vi "Write Report.vi"(8 "error in (no error)":errorcluster, 10 "Resource In":variant, 11 "Analyze Parameter Spectral Calibration in":refnum<class "Analyze Parameter Spectral Calibration.lvclass">) -> (0 "error out":errorcluster, 2 "Resource Out":variant, 3 "Analyze Parameter Spectral Calibration out":refnum<class "Analyze Parameter Spectral Calibration.lvclass">)   [LabVIEW 2020, in "Analyze Parameter Spectral Calibration.lvclass"]
uses:
  Analyze Parameter Spectral Calibration.lvclass
  C:/POLARIS Programme/POLARIS-AS-3-Cams/Submodules/HIJ Vision/Analyze/Analyze Parameter/Analyze Parameter Base/Analyze Parameter Base.lvclass
  <vilib>/Utility/config.llb/Config Data RefNum.ctl
  Analyze Parameter Spectral Calibration.lvclass/Analyze Parameter Spectral Calibration.ctl
  <vilib>/Utility/config.llb/Write Key (Double).vi
  <vilib>/Utility/config.llb/NI_LVConfig.lvlib
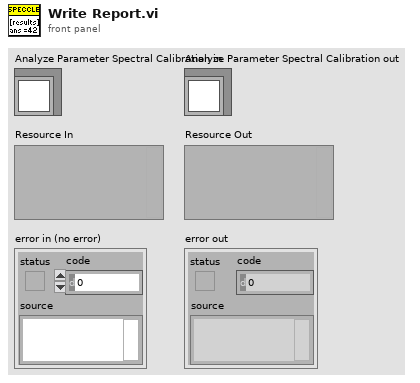
[diagram p1: front panel]
types:
  T1 = typedef "NI_LVConfig.lvlib/Config Data RefNum.ctl" = refnum<k1>
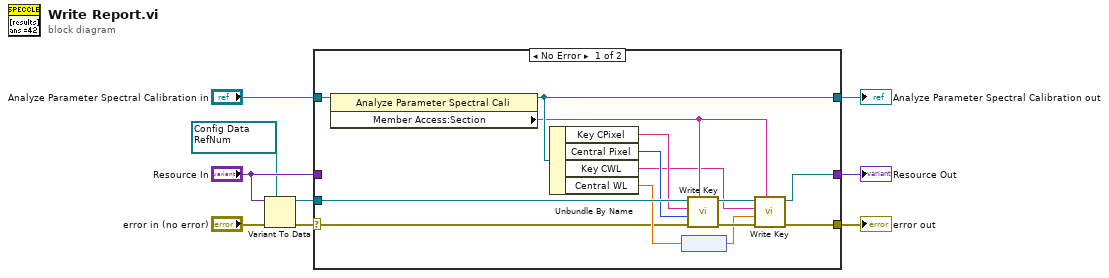
[diagram p0: block diagram]
diagram:
  w6 = T1 refnum items=["config data"] ("refnum")
  n1 = Variant To Data(error in="error in (no error)", type=w6, Variant="Resource In") -> (data=w8:T1, error out=w9:errorcluster)
  n2 = case shown="No Error" w9 {
    selector: w9 -> [w10 w25]
    tunnel: w8 -> [w23 _]
    tunnel: "Analyze Parameter Spectral Calibration in" -> [w22 w24]
    tunnel: [w21 w24] -> w1
    tunnel: [w18 w26] -> w3
    tunnel: [w17 w25] -> w2
    tunnel: "Resource In" -> [_ w26]
    frame No Error {
      n3 = property class="Analyze Parameter Spectral Cali"(reference=w22) -> (reference out=w21:refnum<class "Analyze Parameter Spectral Calibration.lvclass">, "Member Access:Section"=w16:string)  [unwired: 1 in, 1 out]
      n4 = Unbundle By Name(w21) -> ("Key CPixel"=w20:string, "Central Pixel"=w19:i32, "Key CWL"=w13:string, "Central WL"=w12:dbl[unit])
      n5 = node(w12) -> (w11:dbl)
      n6 = call-poly <vilib>:"Write Key.vi"("section"=w16, "error in (no error)"=w10, "value"=w19, "key"=w20, "refnum"=w23) -> ("error out"=w15:errorcluster, "refnum out"=w14:T1)  [unwired: 4 in, 1 out]
      n7 = call-poly <vilib>:"Write Key.vi"("section"=w16, "error in (no error)"=w15, "value"=w11, "key"=w13, "refnum"=w14) -> ("error out"=w17:errorcluster, "refnum out"=w18:T1)  [unwired: 4 in, 1 out]
    }
    frame Error {
    }
  }
  "error out" <- w2
  "Analyze Parameter Spectral Calibration out" <- w1
  "Resource Out" <- w3
